vi "Expt9 niUSRP EX PSK Rx student.vi"() -> ()   [LabVIEW 2020]
doc: "This example <B>requires the Modulation Toolkit</B>.\n\nReceives and demodulates a PSK (Phase Shift Keyed) signal. \n\nThis example is paired with the example \"niUSRP Ex PSK Tx.vi\", which allows you to establish a Tx / Rx link between two separate USRPs. \n\nTo establish a Tx / Rx link between two USRPs:\n1) Ensure that both the Tx and Rx example VIs have matching parameters for Modulation Scheme (M-Ary), Carrier Frequency, and Symbol Rate. Specify the Symbol Rate by setting the combination of the IQ Sampling Rate and the Number of Samples per Symbol parameters.\n2) Choose an IQ Sample Rate that enables sufficient Rx bandwidth.\n3) Set the Tx and / or Rx gain to ensure a sufficient signal to noise ratio on the Receive side. \nNote: applying too much gain can result in clipping.\n4) Choose a sufficient acquisition frame length that enables the demodulator to lock to the transmitted signal. National Instruments recommends that the acquired frame contain a number of symbols that is at least 20 * M-Ary of the modulation scheme. \n5) Ensure that the Reset Demodulator control is set to True until a solid lock is established. \n6) Install antennas and attenuators that efficiently operate at the carrier frequency you choose."
uses:
  <vilib>/addons/Modulation/Analog/support/mod_Set Error Source.vi
  <vilib>/addons/Modulation/Analog/support/Validators/mod_Fractional Resample Validate.vi
  <vilib>/addons/Modulation/Analog/support/Validators/mod_Check Flush State.vi
  <vilib>/addons/Modulation/Analog/support/mod_FractionalResampler.vi
  <vilib>/addons/Modulation/Analog/support/mod_Integer Rate Interpolation.vi
  <vilib>/addons/Modulation/Analog/support/Validators/mod_Validate Complex Waveform.vi
  <vilib>/addons/Modulation/Analog/support/mod_PerformResampling.vi
  <vilib>/addons/Modulation/Analog/support/Validators/mod_WFErrorHandler.vi
  <vilib>/addons/Modulation/Digital/General/MT Generate PSK System Parameters(M).vi
  <vilib>/addons/Modulation/Digital/Support/Common/Validators/mod_Generate Filter Coefficients Validate.vi
  <vilib>/addons/Modulation/Digital/General/subVIs/mod_Generate Filter Coefficients.vi
  <instrlib>/niUSRP/niUSRP Fetch Rx Data (CDB Cluster).vi
  <vilib>/Utility/error.llb/Error Cluster From Error Code.vi
  <vilib>/addons/Modulation/Analog/support/mod_Resampling Factors.vi
  <vilib>/addons/Modulation/Analog/support/mod_ResamplingFilter.vi
  <vilib>/addons/Modulation/Analog/support/mod_Generate Integer Interpolation Filter.vi
  <vilib>/addons/Modulation/niDMT.lvlib
  <vilib>/addons/Modulation/niAMT.lvlib
panel:
  out "error out":errorcluster
  in  "Enabled Channel":string(combo)="0"
  out "Gain [dB] (actual)":dbl=12.0 format="%#.6p"
  out "Carrier Frequency \n[Hz] (actual)":dbl=915000000.0 format="%#.6p"
  out "IQ Sampling\nRate [S/sec] (actual)":dbl=500000.0 format="%#.6p"
  in  "Active Antenna":string(combo)="RX1"
  in  "Gain [dB]":dbl=12.0 format="%#.6p"
  in  "Carrier\nFrequency [Hz]":dbl=915000000.0 format="%#.6p"
  in  "IQ Sampling\nRate [S/sec]":dbl=500000.0 format="%#.6p"
  in  "Device Name":refnum<k15>="192.168.10.4"
  in  "Autoscale":bool
  out "Constellation Graph":T1(graph)
  out "Measurements":T2={"frequency offset (Hz)"=-11.93165072236316, "frequency drift (Hz)"=0.08770196207837619, "phase offset (deg)"=52.673364140832604} {"phase offset (deg)" format="%.2f"; "frequency drift (Hz)" format="%.2f"; "frequency offset (Hz)" format="%.2f"}
  in  "Reset? (t)":bool=TRUE caption="Reset\nDemodulator?"
  in  "Choose a PSK Format":T3(tab)=enum."8-PSK" caption="PSK"
  in  "BPSK System Parameters":T4={"Samples per Symbol"=8, "symbol map"=[], "Differential PSK"=enum."disable", "PSK type"=0} {"PSK type" items=["normal", "shifted", "offset"]; "symbol map" format="%.3f"}
  in  "QPSK System Parameters":T4={"Samples per Symbol"=8, "symbol map"=[], "Differential PSK"=enum."disable", "PSK type"=0} {"PSK type" items=["normal", "shifted", "offset"]; "symbol map" format="%.3f"}
  in  "pi/4 DQPSK System Parameters":T4={"Samples per Symbol"=8, "symbol map"=[], "Differential PSK"=enum."enable", "PSK type"=1} {"PSK type" items=["normal", "shifted", "offset"]; "symbol map" format="%.3f"}
  in  "OQPSK System Parameters":T4={"Samples per Symbol"=8, "symbol map"=[], "Differential PSK"=enum."disable", "PSK type"=2} {"PSK type" items=["normal", "shifted", "offset"]; "symbol map" format="%.3f"}
  in  "8-PSK System Parameters":T4={"Samples per Symbol"=4, "symbol map"=[], "Differential PSK"=enum."disable", "PSK type"=0} {"PSK type" items=["normal", "shifted", "offset"]; "symbol map" format="%.3f"}
  in  "16-PSK System Parameters":T4={"Samples per Symbol"=8, "symbol map"=[], "Differential PSK"=enum."disable", "PSK type"=0} {"PSK type" items=["normal", "shifted", "offset"]; "symbol map" format="%.3f"}
  in  "M":i32=4 min=2 step=2
  in  "Custom System Parameters":T4={"Samples per Symbol"=8, "symbol map"=[], "Differential PSK"=enum."disable", "PSK type"=0} {"PSK type" items=["normal", "shifted", "offset"]; "symbol map" format="%.3f"}
  in  "Filter Parameters":T5={"Alpha"=0.5, "Filter Length"=6, "TX Filter"=enum."Root Raised Cos"} {"Alpha" format="%.2f"}
  out "Symbol Rate [Hz]":dbl=125000.0 caption="Symbol Rate, \n[symbols/sec]" format="%.2p"
  out "Frame Size [samples]":i64=20000
  in  "Acq Duration [sec]":dbl=0.01 format="%#.6p"
  in  "Stop":bool
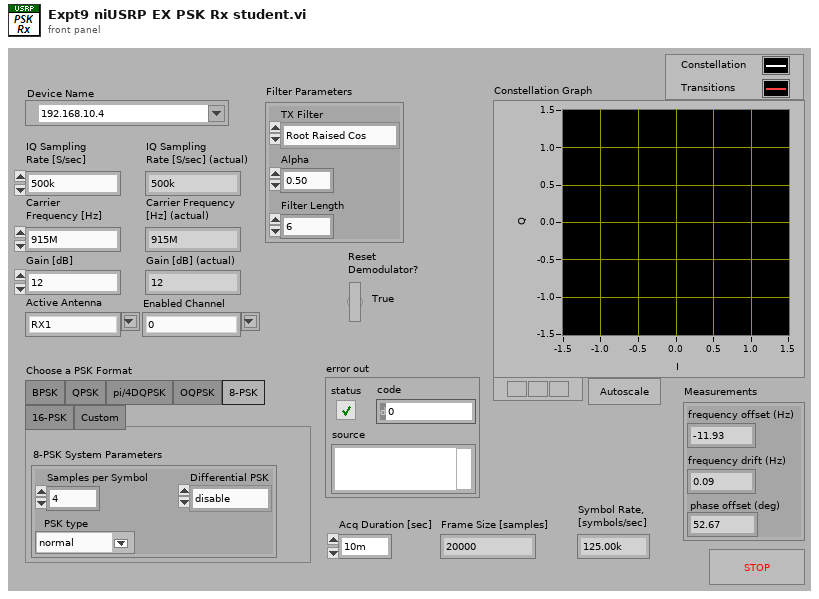
[diagram p1: front panel]
types:
  T1 = cluster{"Decimated Array":dbl[], "Decimated Array":dbl[]}[]
  T2 = cluster{"frequency offset (Hz)":dbl, "frequency drift (Hz)":dbl, "phase offset (deg)":dbl}
  T3 = enum32{"BPSK", "QPSK", "pi/4DQPSK", "OQPSK", "8-PSK", "16-PSK", "Custom"}
  T4 = cluster{"Samples per Symbol":i32, "symbol map":cdb[], "Differential PSK":enum16{"disable", "enable"}, "PSK type":u16}
  T5 = cluster{"Alpha":dbl, "Filter Length":i32, "TX Filter":enum16{"none", "Raised Cosine", "Root Raised Cos", "Gaussian"}}
  T6 = enum16{"FSK", "PSK", "QAM", "MSK", "PAM", "ASK", "CPM"}
  T7 = enum16{"none", "Raised Cosine", "Root Raised Cos", "Gaussian"}
  T8 = cluster{"samples per symbol (16)":i32, "symbol map":cdb[], "differential PSK":enum16{"disable", "enable"}, "PSK type":u16}
  T9 = typedef "niAMT.lvlib/Complex Data Waveform.ctl" = cluster{"t0":dbl, "dt":dbl, "Y":cdb[]}
  T10 = cluster{"constellation":dbl[], "oversampled data":dbl[]}[]
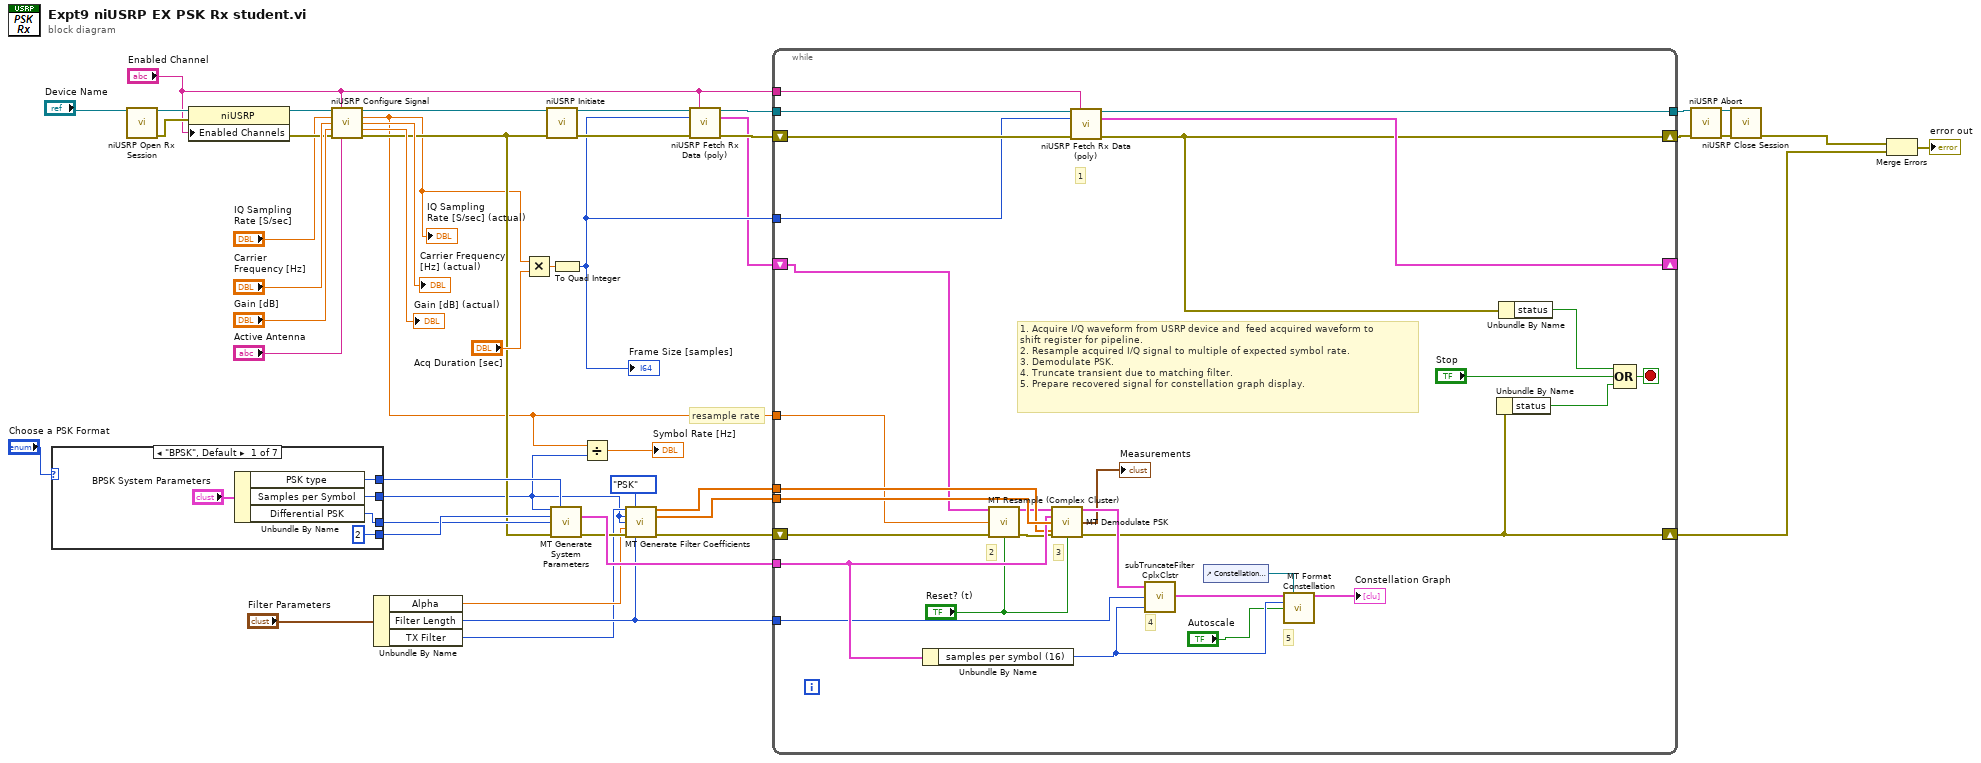
[diagram p0: block diagram]
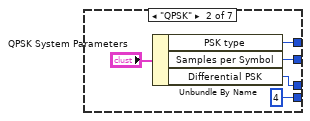
[diagram p2: hidden frame]
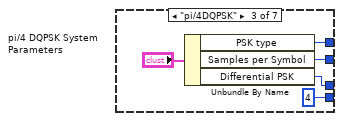
[diagram p3: hidden frame]
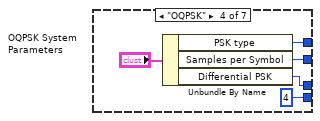
[diagram p4: hidden frame]
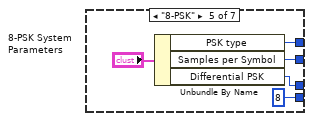
[diagram p5: hidden frame]
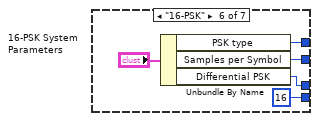
[diagram p6: hidden frame]
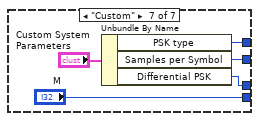
[diagram p7: hidden frame]
diagram:
  # "resample rate"
  n1 = case shown="\"BPSK\", Default" "Choose a PSK Format" {
    tunnel: [w49 w55 w60 w65 w70 w76 w80] -> w4
    tunnel: [w47 w52 w57 w62 w67 w72 w77] -> w34
    tunnel: [2 ("M-PSK (4)") 4 ("M-PSK (4)") 4 ("M-PSK (4)") 4 ("M-PSK (4)") 8 ("M-PSK (4)") 16 ("M-PSK (4)") "M"] -> w35
    tunnel: [w50 w54 w59 w64 w71 w74 w81] -> w33
    frame "BPSK", Default {
      n2 = Unbundle By Name("BPSK System Parameters") -> ("PSK type"=w50:u16, "Samples per Symbol"=w49:i32, "Differential PSK"=w47:enum16{"disable", "enable"})
    }
    frame "QPSK" {
      n3 = Unbundle By Name("QPSK System Parameters") -> ("PSK type"=w54:u16, "Samples per Symbol"=w55:i32, "Differential PSK"=w52:enum16{"disable", "enable"})
    }
    frame "pi/4DQPSK" {
      n4 = Unbundle By Name("pi/4 DQPSK System Parameters") -> ("PSK type"=w59:u16, "Samples per Symbol"=w60:i32, "Differential PSK"=w57:enum16{"disable", "enable"})
    }
    frame "OQPSK" {
      n5 = Unbundle By Name("OQPSK System Parameters") -> ("PSK type"=w64:u16, "Samples per Symbol"=w65:i32, "Differential PSK"=w62:enum16{"disable", "enable"})
    }
    frame "8-PSK" {
      n6 = Unbundle By Name("8-PSK System Parameters") -> ("PSK type"=w71:u16, "Samples per Symbol"=w70:i32, "Differential PSK"=w67:enum16{"disable", "enable"})
    }
    frame "16-PSK" {
      n7 = Unbundle By Name("16-PSK System Parameters") -> ("PSK type"=w74:u16, "Samples per Symbol"=w76:i32, "Differential PSK"=w72:enum16{"disable", "enable"})
    }
    frame "Custom" {
      n8 = Unbundle By Name("Custom System Parameters") -> ("PSK type"=w81:u16, "Samples per Symbol"=w80:i32, "Differential PSK"=w77:enum16{"disable", "enable"})
    }
  }
  n9 = call <instrlib>:"niUSRP Open Rx Session.vi"("device names"="Device Name") -> ("session handle out"=w10:refnum<k15>, "error out"=w9:errorcluster)  [unwired: 13 in]
  n10 = property class="niUSRP"(reference=w10, error in=w9, "Enabled Channels"="Enabled Channel") -> (reference out=w8:refnum<k15>, error out=w7:errorcluster)
  n11 = call <instrlib>:"niUSRP Configure Signal.vi"("session handle"=w8, "channel list"="Enabled Channel", "IQ rate"="IQ Sampling\nRate [S/sec]", "carrier frequency"="Carrier\nFrequency [Hz]", "gain"="Gain [dB]", "error in (no error)"=w7, "active antenna"="Active Antenna") -> ("session handle out"=w20:refnum<k15>, "coerced IQ rate"=w2:dbl, "coerced carrier frequency"=→"Carrier Frequency \n[Hz] (actual)":dbl, "coerced gain"=→"Gain [dB] (actual)":dbl, "error out"=w19:errorcluster)  [unwired: 4 in]
  "IQ Sampling\nRate [S/sec] (actual)" <- w2
  n12 = Unbundle By Name("Filter Parameters") -> ("Alpha"=w38:dbl, "Filter Length"=w37:i32, "TX Filter"=w36:T7)
  n13 = Multiply(x=w2, y="Acq Duration [sec]") -> (x*y=w45:dbl)
  n14 = call <instrlib>:"niUSRP Initiate.vi"("session handle"=w20, "error in (no error)"=w19) -> ("session handle out"=w18:refnum<k15>, "error out"=w17:errorcluster)  [unwired: 12 in]
  n15 = call-poly <vilib>:"MT Generate System Parameters.vi"("samples per symbol (16)"=w4, "PSK type"=w33, "M-PSK (4)"=w35, "differential PSK"=w34, "error in (no error)"=w19) -> ("PSK system parameters"=w41:T8, "error out"=w40:errorcluster)  [unwired: 8 in, 1 out]
  n16 = To Quad Integer(1:w45) -> (0:w16:i64)
  "Frame Size [samples]" <- w16
  n17 = Divide(x=w2, y=w4) -> (x/y=→"Symbol Rate [Hz]":dbl)
  n18 = call <vilib>:"MT Generate Filter Coefficients.vi"("pulse shaping filter (none)"=w36, "modulation type"=T6."PSK", "pulse shaping samples per symbol (16)"=w4, "matched samples per symbol (16)"=w4, "filter parameter"=w38, "error in (no error)"=w40, "filter length (symbols)"=w37) -> ("pulse shaping filter coefficients"=w31:dbl[], "matched filter coefficients"=w42:dbl[], "error out"=w43:errorcluster)  [unwired: 6 in]
  n19 = call-poly <instrlib>:"niUSRP Fetch Rx Data (poly).vi"("session handle"=w18, "channel list"="Enabled Channel", "number of samples"=w16, "error in (no error)"=w17) -> ("session handle out"=w14:refnum<k15>, "data"=w13:cluster{"t0":dbl, "dt":dbl, "Y":cdb[]}, "error out"=w15:errorcluster)  [unwired: 8 in, 1 out]
  n20 = while {
    tunnel: [w97] -> w27
    shift-right: [w94] -> w28
    shift-left: w15 -> [w98]
    shift-right: [w104] -> w11
    shift-left: w43 -> [w90]
    tunnel: w16 -> [w96]
    tunnel: w14 -> [w99]
    tunnel: w42 -> [w108]
    tunnel: w41 -> [w107]
    tunnel: w2 -> [w91]
    tunnel: w37 -> [w106]
    tunnel: w31 -> [w101]
    shift-right: [w95] -> _
    shift-left: w13 -> [w92]
    tunnel: "Enabled Channel" -> [w93]
    stop <- w110 stop-if-true
    # "5"
    # "4"
    # "3"
    # "2"
    # "1"
    # "1. Acquire I/Q waveform from USRP device and  feed acquired waveform to\nshift register for pipeline.\n2. Resample acquired I/Q signal to multiple of expected symbol rate.\n3. Demodulate PSK.\n4. Truncate transient due to matching filter.\n5. Prepare recovered signal for constellation graph display."
    n21 = Unbundle By Name(w107) -> ("samples per symbol (16)"=w83:i32)
    n22 = call <vilib>:"MT Resample (Complex Cluster).vi"("input complex waveform"=w92, "desired sample rate (Hz)"=w91, "error in (no error)"=w90, "reset? (T)"="Reset? (t)") -> ("output complex waveform"=w88:T9, "error out"=w89:errorcluster)  [unwired: 10 in]
    n23 = call <vilib>:"MT Demodulate PSK.vi"("input complex waveform"=w88, "PSK system parameters"=w107, "matched filter coefficients"=w108, "error in (no error)"=w89, "pulse shaping filter coefficients"=w101, "reset? (T)"="Reset? (t)") -> ("recovered complex waveform"=w105:T9, "measurements"=→"Measurements":T2, "error out"=w104:errorcluster)  [unwired: 5 in, 2 out]
    n24 = call-poly <instrlib>:"niUSRP Fetch Rx Data (poly).vi"("session handle"=w99, "channel list"=w93, "number of samples"=w96, "error in (no error)"=w98) -> ("session handle out"=w97:refnum<k15>, "data"=w95:cluster{"t0":dbl, "dt":dbl, "Y":cdb[]}, "error out"=w94:errorcluster)  [unwired: 8 in, 1 out]
    n25 = call "subTruncateFilterCplxClstr.vi"("samples per symbol (16)"=w83, "filter length (symbols)"=w106, "waveform to truncate"=w105) -> ("truncated waveform"=w84:T9)
    n26 = control-ref of="Constellation Graph"() -> (w86:refnum<vi>)
    n27 = call <vilib>:"MT Format Constellation.vi"("waveform"=w84, "constellation reference"=w86, "samples per symbol"=w83, "autoscale"="Autoscale") -> ("constellation graph"=→"Constellation Graph":T10)  [unwired: 10 in, 1 out]
    n28 = Unbundle By Name(w104) -> ("status"=w102:bool)
    n29 = Unbundle By Name(w94) -> ("status"=w109:bool)
    n30 = Compound Arithmetic op=OR(w109, "Stop", w102) -> (w110:bool)
  }
  n31 = call <instrlib>:"niUSRP Abort.vi"("session handle"=w27, "error in (no error)"=w28) -> ("session handle out"=w30:refnum<k15>, "error out"=w29:errorcluster)  [unwired: 12 in]
  n32 = call <instrlib>:"niUSRP Close Session.vi"("session handle"=w30, "error in (no error)"=w29) -> ("error out"=w12:errorcluster)  [unwired: 13 in]
  n33 = Merge Errors(w12, w11) -> (→"error out":errorcluster)
